vi "graph_xy.vi"() -> ()   [LabVIEW 2020]
uses:
  <vilib>/Analysis/1siggen.llb/Ramp Pattern by Samples.vi
  <vilib>/Analysis/NI_AALBase.lvlib
panel:
  out "graph":T1(graph)
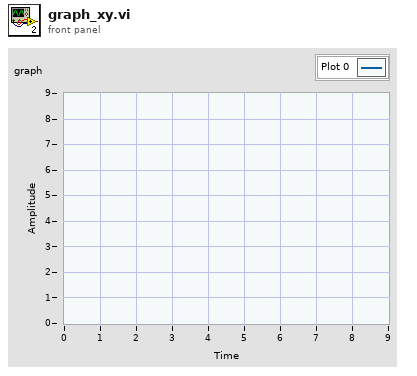
[diagram p1: front panel]
types:
  T1 = cluster{"Ramp Pattern":dbl[], "Ramp Pattern":dbl[]}
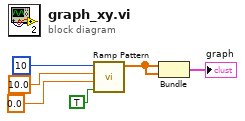
[diagram p0: block diagram]
diagram:
  n1 = call-poly <vilib>:"Ramp Pattern.vi"("exclude end?"=TRUE, "start"=0.0, "end"=10.0, "samples"=10) -> ("Ramp Pattern"=w2:dbl[])  [unwired: 6 in, 1 out]
  n2 = Bundle("Ramp Pattern"=w2, "Ramp Pattern"=w2) -> (→"graph":T1)  [unwired: 1 in]
